vi "FFXCKI.VI"() -> (0 "XCKactive":u8)   [LabVIEW 2015]
uses:
  ESLSCDLL.dll
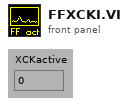
[diagram p1: front panel]
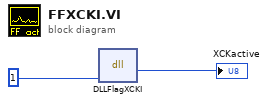
[diagram p0: block diagram]
diagram:
  n1 = dll-call lib="C:/ENTW/PCIE/64bit/lv64/1cam/board.vis/ESLSCDLL.dll" fn="DLLFlagXCKI"("drv"=u32 1) -> ("Rückgabetyp"=→"XCKactive":u8)  [unwired: 4 in, 2 out]
